vi "SetTemp.vi"(1 "Error In":errorcluster, 2 "Numeric Control":dbl) -> (0 "Error Out":errorcluster)   [LabVIEW 2014]
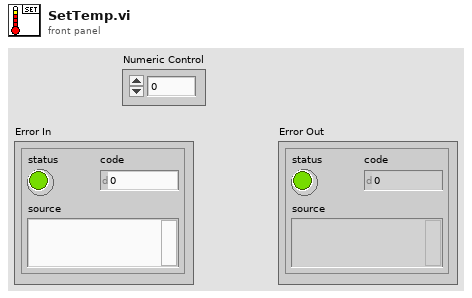
[diagram p1: front panel]
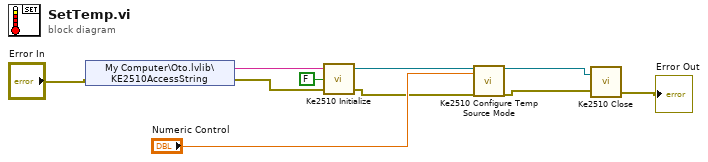
[diagram p0: block diagram]
diagram:
  n1 = shared-variable "My Computer\\Oto.lvlib\\KE2510AccessString"(error in="Error In") -> (w10:string, error out=w9:errorcluster)
  n2 = call <instrlib>:"Ke2510 Initialize.vi"("error in (no error)"=w9, "reset device"=FALSE, "resource name"=w10) -> ("error out"=w6:errorcluster, "instrument handle"=w7:refnum<visa-resource-name>)  [unwired: 1 out]
  n3 = call <instrlib>:"Ke2510 Configure Temp Source Mode.vi"("instrument handle"=w7, "setpoint"="Numeric Control", "error in (no error)"=w6) -> ("instrument handle out"=w5:refnum<visa-resource-name>, "error out"=w4:errorcluster)  [unwired: 14 in, 1 out]
  n4 = call <instrlib>:"Ke2510 Close.vi"("instrument handle"=w5, "error in (no error)"=w4) -> ("error out"=→"Error Out":errorcluster)  [unwired: 1 in, 1 out]
